vi "updateColumnHeaders.vi"(8 "error in (no error)":errorcluster, 11 "InputDataLogger in":refnum<class "StiffnessLog.lvclass">) -> (0 "error out":errorcluster, 3 "InputDataLogger out":refnum<class "StiffnessLog.lvclass">)   [LabVIEW 2013, in "StiffnessLog.lvclass"]
uses:
  StiffnessLog.lvclass
  <userlib>/Common/Log/Log/Log.lvclass/Log.ctl
  <userlib>/Common/Log/Log/Log.lvclass
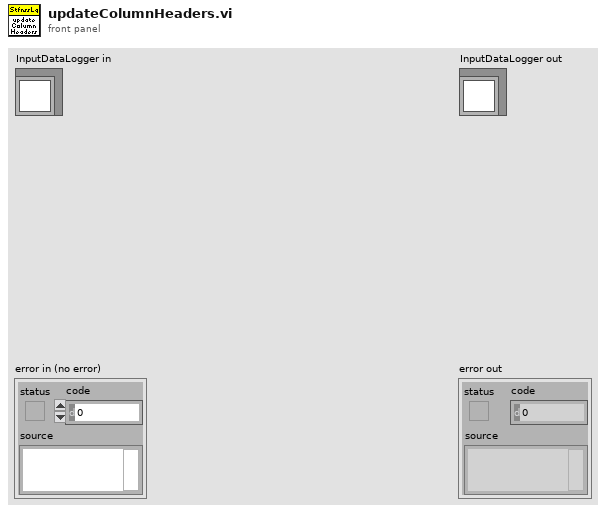
[diagram p1: front panel]
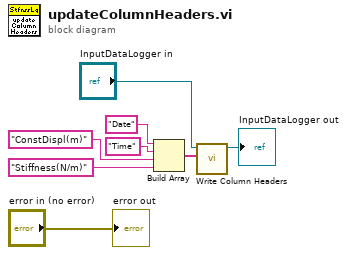
[diagram p0: block diagram]
diagram:
  n1 = Build Array("Date" ("element"), "Time", "ConstDispl(m)", "Stiffness(N/m)") -> (w5:string[])
  n2 = call <userlib>:"Write Column Headers.vi"("Column Headers"=w5, "Logger in"="InputDataLogger in") -> ("Logger out"=→"InputDataLogger out":refnum<class "StiffnessLog.lvclass">)  [unwired: 9 in]
  "error out" <- "error in (no error)"
